vi "Umgebung.Aussentemperatur.vi"(8 "Error in":errorcluster, 11 "Umgebung in":refnum<data-value>) -> (0 "Error out":errorcluster, 3 "Umgebung out":refnum<data-value>)   [LabVIEW 2016, in "Umgebung.lvclass"]
uses:
  Umgebung.lvclass
  Umgebung.lvclass/Umgebung.ctl
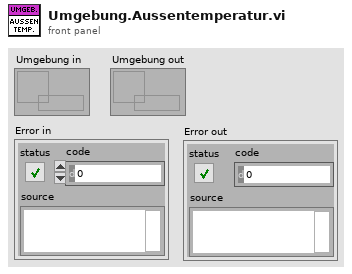
[diagram p1: front panel]
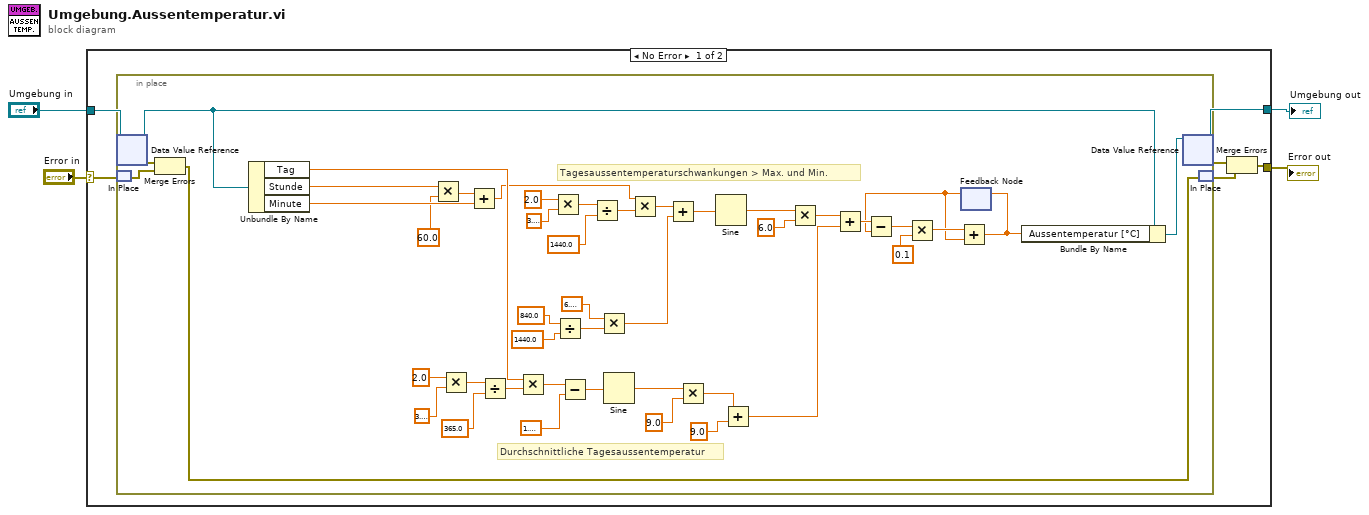
[diagram p0: block diagram]
diagram:
  n1 = case shown="No Error" "Error in" {
    selector: "Error in" -> [w7 w57]
    tunnel: [w8 w57] -> w2
    tunnel: [w10 w56] -> w3
    tunnel: "Umgebung in" -> [w5 w56]
    frame No Error {
      n2 = in-place {
        # "Tagesaussentemperaturschwankungen > Max. und Min."
        # "Durchschnittliche Tagesaussentemperatur"
        n3 = in-place-dvr #1(w5) -> (w51:refnum<class "Umgebung.lvclass">, w53:errorcluster)
        n4 = in-place-match #2(w7) -> (w52:errorcluster)
        n5 = Merge Errors(w53, w52) -> (w55:errorcluster)
        n6 = Unbundle By Name(w51) -> ("Tag"=w54:dbl, "Stunde"=w49:dbl, "Minute"=w48:dbl)
        n7 = Multiply(x=w49, y=60.0) -> (x*y=w16:dbl)
        n8 = Multiply(x=2.0, y=3.141592653589793) -> (x*y=w40:dbl)
        n9 = Add(x=w16, y=w48) -> (x+y=w17:dbl)
        n10 = Divide(x=w40, y=365.0) -> (x/y=w38:dbl)
        n11 = Multiply(x=w54, y=w38) -> (x*y=w37:dbl)
        n12 = Multiply(x=2.0, y=3.141592653589793) -> (x*y=w29:dbl)
        n13 = Divide(x=840.0 ("y"), y=1440.0) -> (x/y=w21:dbl)
        n14 = Subtract(x=w37, y=1.5707963267948966) -> (x-y=w35:dbl)
        n15 = Divide(x=w29, y=1440.0) -> (x/y=w27:dbl)
        n16 = Multiply(x=6.283185307179586, y=w21) -> (x*y=w20:dbl)
        n17 = Sine(x=w35) -> (sin(x)=w43:dbl)
        n18 = Multiply(x=w17, y=w27) -> (x*y=w25:dbl)
        n19 = Add(x=w25, y=w20) -> (x+y=w26:dbl)
        n20 = Multiply(x=w43, y=9.0) -> (x*y=w45:dbl)
        n21 = Sine(x=w26) -> (sin(x)=w32:dbl)
        n22 = Add(x=w45, y=9.0) -> (x+y=w19:dbl)
        n23 = Multiply(x=w32, y=6.0) -> (x*y=w34:dbl)
        n24 = Add(x=w34, y=w19) -> (x+y=w13:dbl)
        n25 = feedback #3() -> (w11:dbl)  [unwired: 1 in]
        n26 = Subtract(x=w13, y=w11) -> (x-y=w14:dbl)
        n27 = Multiply(x=w14, y=0.1) -> (x*y=w15:dbl)
        n28 = Add(x=w15, y=w11) -> (x+y=w47:dbl)
        n29 = feedback-in #3(w47) -> ()
        n30 = Bundle By Name(cluster=w51, "Aussentemperatur [°C]"=w47) -> (w50:refnum<class "Umgebung.lvclass">)
        n31 = in-place-dvr #1(w50) -> (w10:refnum<data-value>, w9:errorcluster)
        n32 = in-place-match #2(w55) -> (w6:errorcluster)
      }
      n33 = Merge Errors(w9, w6) -> (w8:errorcluster)
    }
    frame Error {
    }
  }
  "Umgebung out" <- w3
  "Error out" <- w2
